vi "Tangent hyperbolic derivative.vi"(1 "x":dbl format="%.2f") -> (0 "y=f(x) d'tan.hyp":dbl format="%.2f")   [LabVIEW 2010]
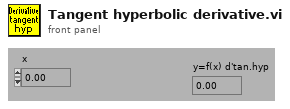
[diagram p1: front panel]
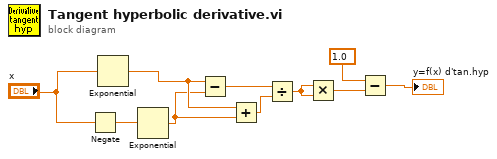
[diagram p0: block diagram]
diagram:
  n1 = Negate(x="x") -> (-x=w9:dbl)
  n2 = Exponential(1:"x") -> (0:w8:dbl)
  n3 = Exponential(1:w9) -> (0:w7:dbl)
  n4 = Subtract(x=w8, y=w7) -> (x-y=w6:dbl)
  n5 = Add(x=w8, y=w7) -> (x+y=w5:dbl)
  n6 = Divide(x=w6, y=w5) -> (x/y=w4:dbl)
  n7 = Multiply(x=w4, y=w4) -> (x*y=w3:dbl)
  n8 = Subtract(x=1.0, y=w3) -> (x-y=→"y=f(x) d'tan.hyp":dbl)
